vi "MUX80_Split_Page_Boolean.vi"(0 "Array In":bool[](array[boolean])) -> (1 "Page 1 out":bool[](array[boolean]), 2 "Page 6 out":bool[](array[boolean]), 3 "Page 2 out":bool[](array[boolean]), 4 "Page 3 out":bool[](array[boolean]), 5 "Page 4 out":bool[](array[boolean]), 6 "Page 5 out":bool[](array[boolean]))   [LabVIEW 2020]
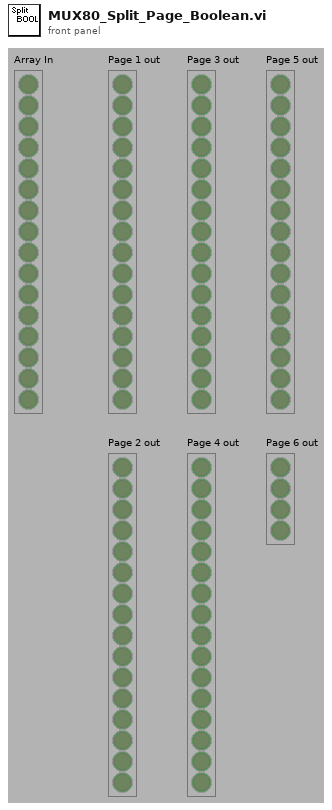
[diagram p1: front panel]
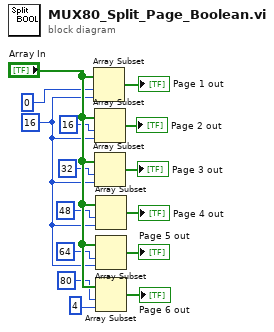
[diagram p0: block diagram]
diagram:
  w7 = 16
  n1 = Array Subset(array="Array In", index=0, length=w7) -> (→"Page 1 out":bool[])
  n2 = Array Subset(array="Array In", index=16, length=w7) -> (→"Page 2 out":bool[])
  n3 = Array Subset(array="Array In", index=32, length=w7) -> (→"Page 3 out":bool[])
  n4 = Array Subset(array="Array In", index=48, length=w7) -> (→"Page 4 out":bool[])
  n5 = Array Subset(array="Array In", index=64, length=w7) -> (→"Page 5 out":bool[])
  n6 = Array Subset(array="Array In", index=80, length=4) -> (→"Page 6 out":bool[])
